vi "Perspective Calibration Example.vi"() -> ()   [LabVIEW 2011]
doc: "Description:\nThis example illustrates the use of a calibration grid to calibrate an image for perspective distortion and converts the locations of features found in the image into the locations in the real world. The example then performs accurate measurements in real world units using these locations.\n\nThis example loads a template image of a grid that is used to calibrate a system, uses the image loaded to learn the calibration from the grid, and measures distances of a distortion template with the learned calibration information."
uses:
  <vilib>/vision/Pattern Matching.llb/IMAQ Curve Parameters.ctl
  <vilib>/vision/Calibration.llb/Error Statistics.ctl
  <vilib>/vision/Calibration.llb/Distortion Model.ctl
  <vilib>/vision/Calibration.llb/Distortion Model Types.ctl
  <vilib>/vision/Clamp.llb/Edge Polarity Type.ctl
  <vilib>/vision/NI_Vision_Development_Module.lvlib
panel:
  out "Part Measurements":T1(array[cluster]) {"Distance (Pixels)" format="%#.2g"; "Distance (Real World)" format="%#.2g"; "Angle (Absolute)" format="%#.2g"; "Angle (Relative)" format="%#_2g"}
  out "Calibration Error Statistics":T2 {"% Distortion" format="%#.6g"; "Standard Deviation" format="%#.6g"; "Mean Error" format="%#.6g"; "Maximum Error" format="%#.6g"}
  in  "Curve Extraction Settings":T3={"Extraction Mode"=0, "Edge Threshold"=40, "Edge Filter Size"=1, "Min Length"=10, "Row Search Step Size"=5, "Col Search Step Size"=5, "Max Endpoint Gap"=5, "Closed"=FALSE, "Subpixel"=FALSE} {"Extraction Mode" items=["Normal", "Uniform Regions"]; "Edge Filter Size" items=["Fine", "Normal", "Contour Tracing"]; "Max Endpoint Gap" min=0; "Col Search Step Size" min=1 max=255 step=1; "Row Search Step Size" min=1 max=255 step=1; "Min Length" min=0; "Edge Threshold" min=1 max=350 step=1}
  in  "Tab Control":T4(tab)
  out "Display 4":T5(plugin-control)
  out "Display 1":T5(plugin-control)
  out "Display 2":T5(plugin-control)
  out "Display 3":T5(plugin-control)
  out "Parts Image Path":path
  out "Calibration Grid Path":path
  # "This example demonstrates how to use a calibration grid to learn the distortion model for a camera and image acquisition setup, and how to learn a perspective calibration using a polynomial model.\n\nThe calibration is used to calibrate an image acquired with the same setup, and then locate and measure parts in the image."
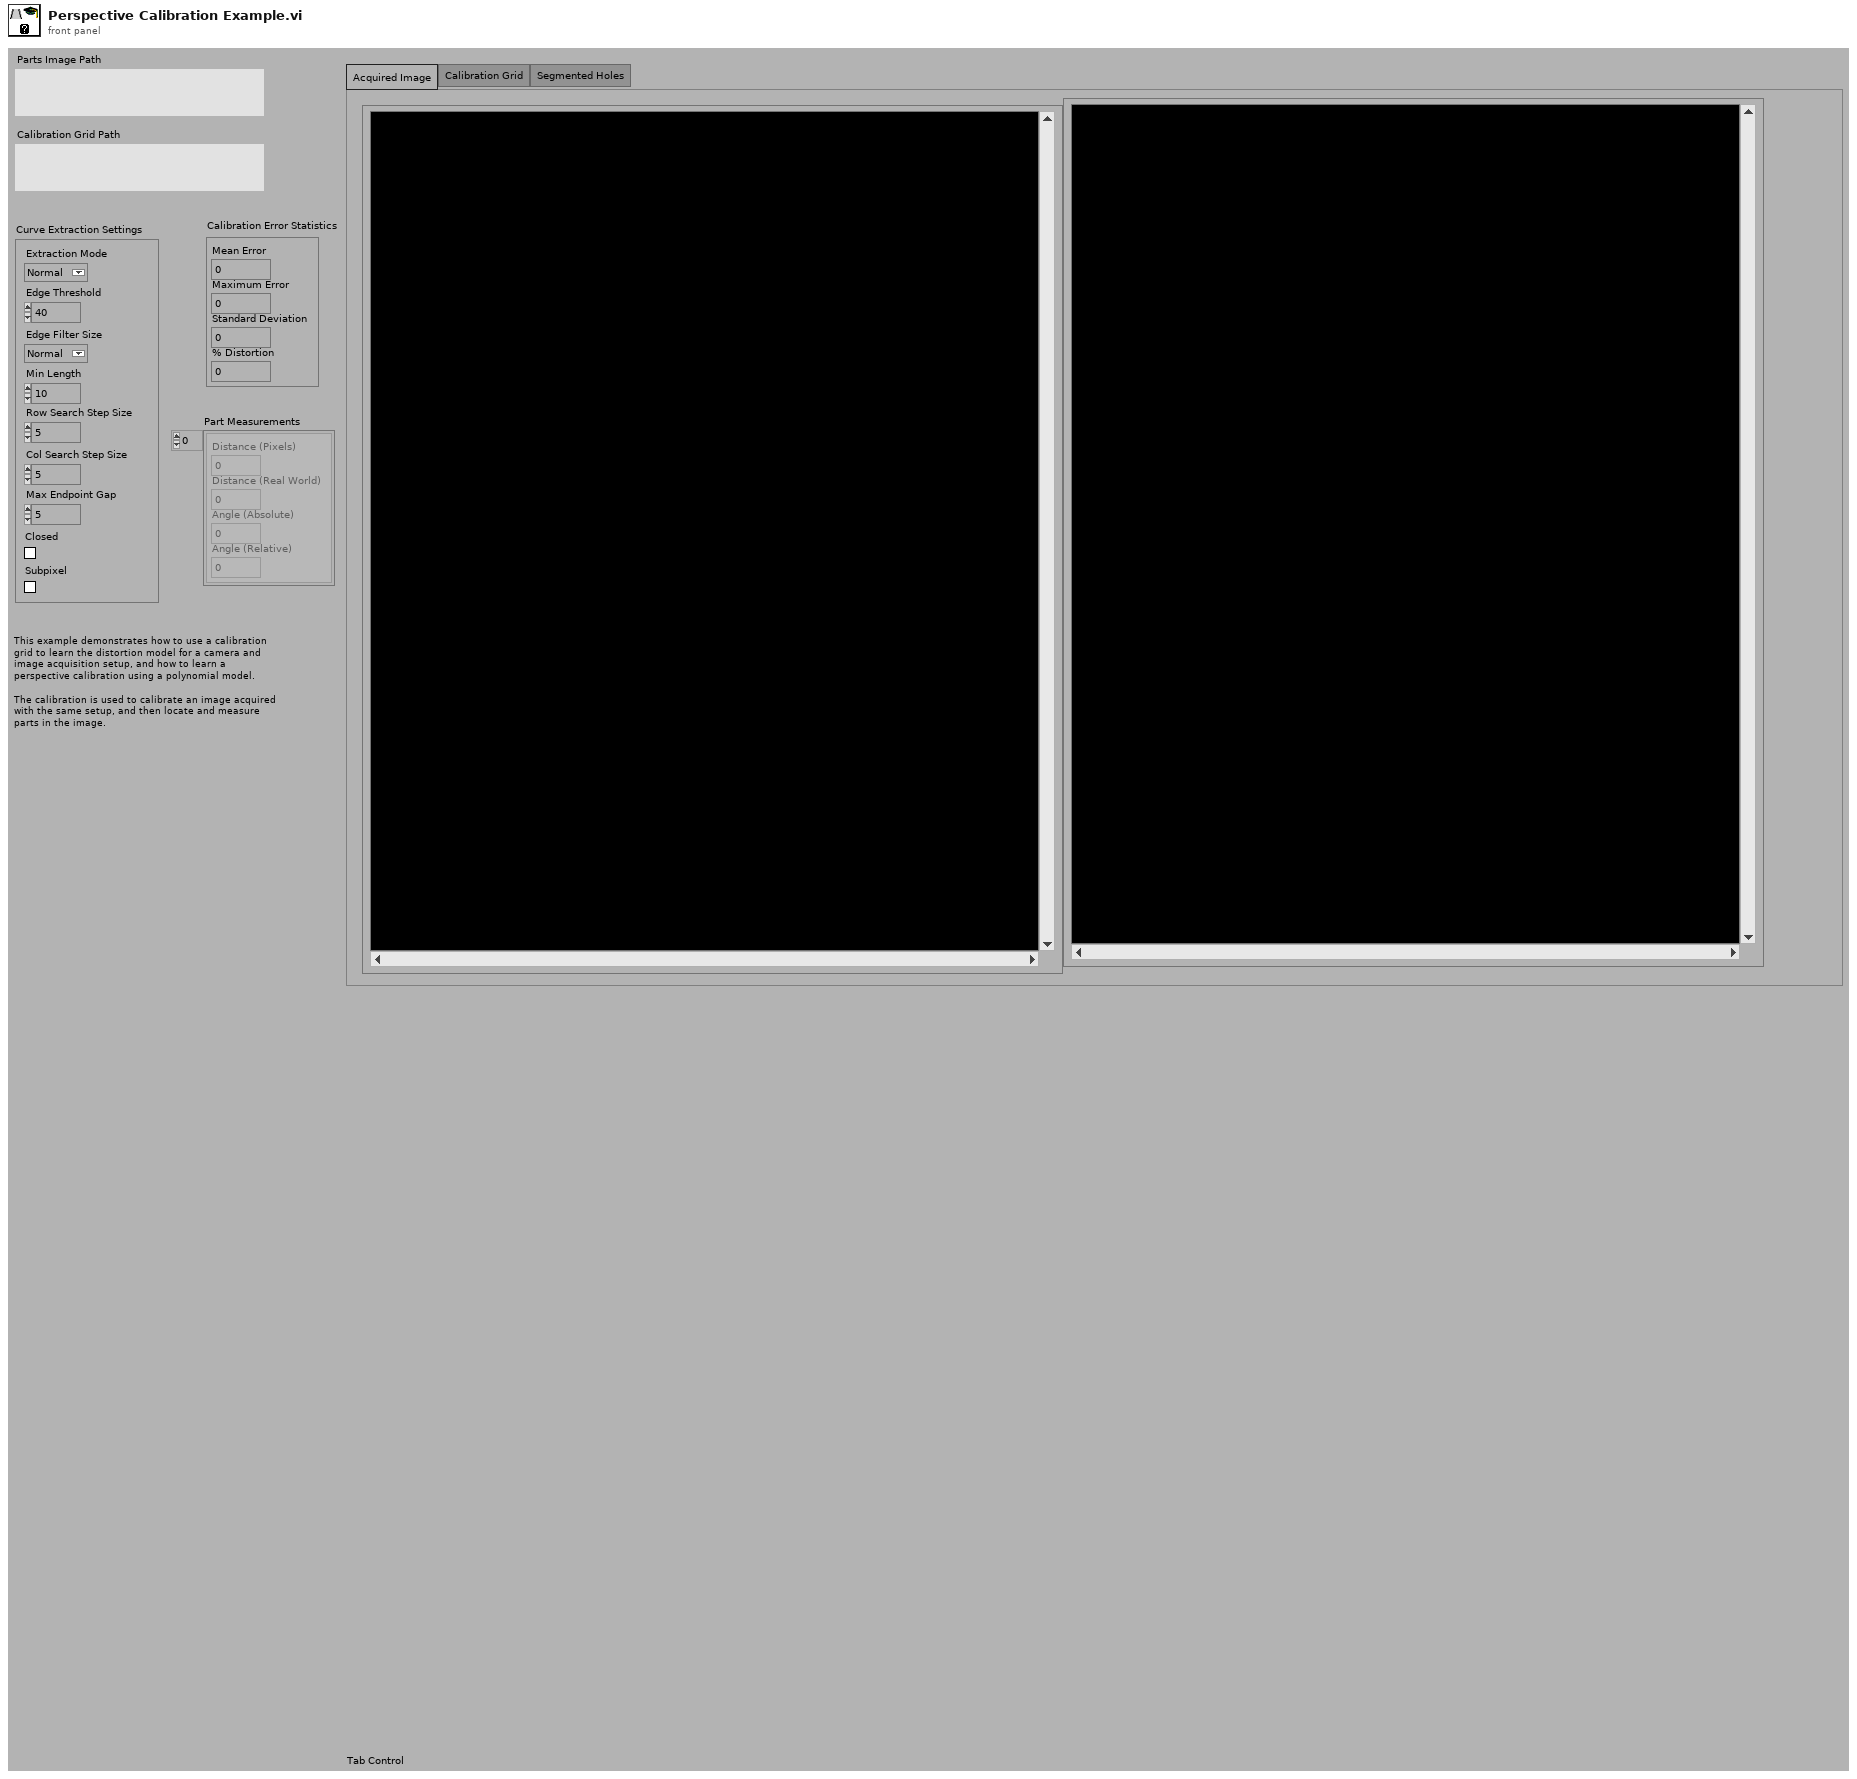
[diagram p1: front panel]
types:
  T1 = cluster{"Distance (Pixels)":dbl, "Distance (Real World)":dbl, "Angle (Absolute)":dbl, "Angle (Relative)":dbl}[]
  T2 = typedef "Error Statistics.ctl" = cluster{"Mean Error":dbl, "Maximum Error":dbl, "Standard Deviation":dbl, "% Distortion":dbl}
  T3 = typedef "IMAQ Curve Parameters.ctl" = cluster{"Extraction Mode":u32, "Edge Threshold":i32, "Edge Filter Size":u32, "Min Length":i32, "Row Search Step Size":i32, "Col Search Step Size":i32, "Max Endpoint Gap":i32, "Closed":bool, "Subpixel":bool}
  T4 = enum32{"Acquired Image", "Calibration Grid", "Segmented Holes"}
  T5 = typedef "IMAQ Image.ctl" = refnum<image>
  T6 = typedef "Distortion Model.ctl" = cluster{"Distortion Model":T7, "Polynomial Model Setup":cluster{"Radial Coefficient":u32, "Tangential Coefficients ":bool}}
  T7 = typedef "Distortion Model Types.ctl" = i32
  T8 = typedef "Particle Parameters" = i32
  T9 = cluster{"Measurement Parameter":T8, "Range Lower Value":dbl, "Range Upper Value":dbl, "Range":bool, "Measurement Type":bool}[]
  T10 = typedef "Image Unit" = enum32{"Undefined", "Angström", "Micrometer", "Millimeter", "Centimeter", "Meter", "Kilometer", "Microinch", "Inch", "Feet", "Nautical miles", "Standard miles", "Steps"}
  T11 = typedef "Calibration Reference Points.ctl" = cluster{"Pixel Coordinates":cluster{"X":dbl, "Y":dbl}[], "Real World Coordinates":cluster{"X":dbl, "Y":dbl}[], "Unit":T10, "Image Size":cluster{"X":u32, "Y":u32}}
  T12 = cluster{"Area":dbl, "Number of Holes":dbl, "Bounding Rect":cluster{"Left":dbl, "Top":dbl, "Right":dbl, "Bottom":dbl}, "Center of Mass":cluster{"X":dbl, "Y":dbl}, "Orientation":dbl, "Dimensions":cluster{"Width":dbl, "Height":dbl}}[]
  T13 = cluster{"Show Search Area":bool, "Show Curves":bool, "Show Clamp Locations":bool, "Show Result":bool, "Search Area Color":u32, "Curves Color":u32, "Clamp Locations Color":u32, "Result Color":u32, "Overlay Group Name":string}
  T14 = typedef "Edge Polarity Type.ctl" = u32
  T15 = cluster{"Angle Range (+/-)":dbl, "Edge Polarity":cluster{"Start":T14, "End":T14}}
  T16 = typedef "ROI Descriptor" = cluster{"Global Rectangle":i32[], "Contours":cluster{"ID":enum32{"External", "Internal"}, "Type":u32, "Coordinates":i32[]}[]}
  T17 = cluster{"Distance (Pixels)":dbl, "Distance (Real World)":dbl, "Angle (Absolute)":dbl, "Angle (Relative)":dbl}
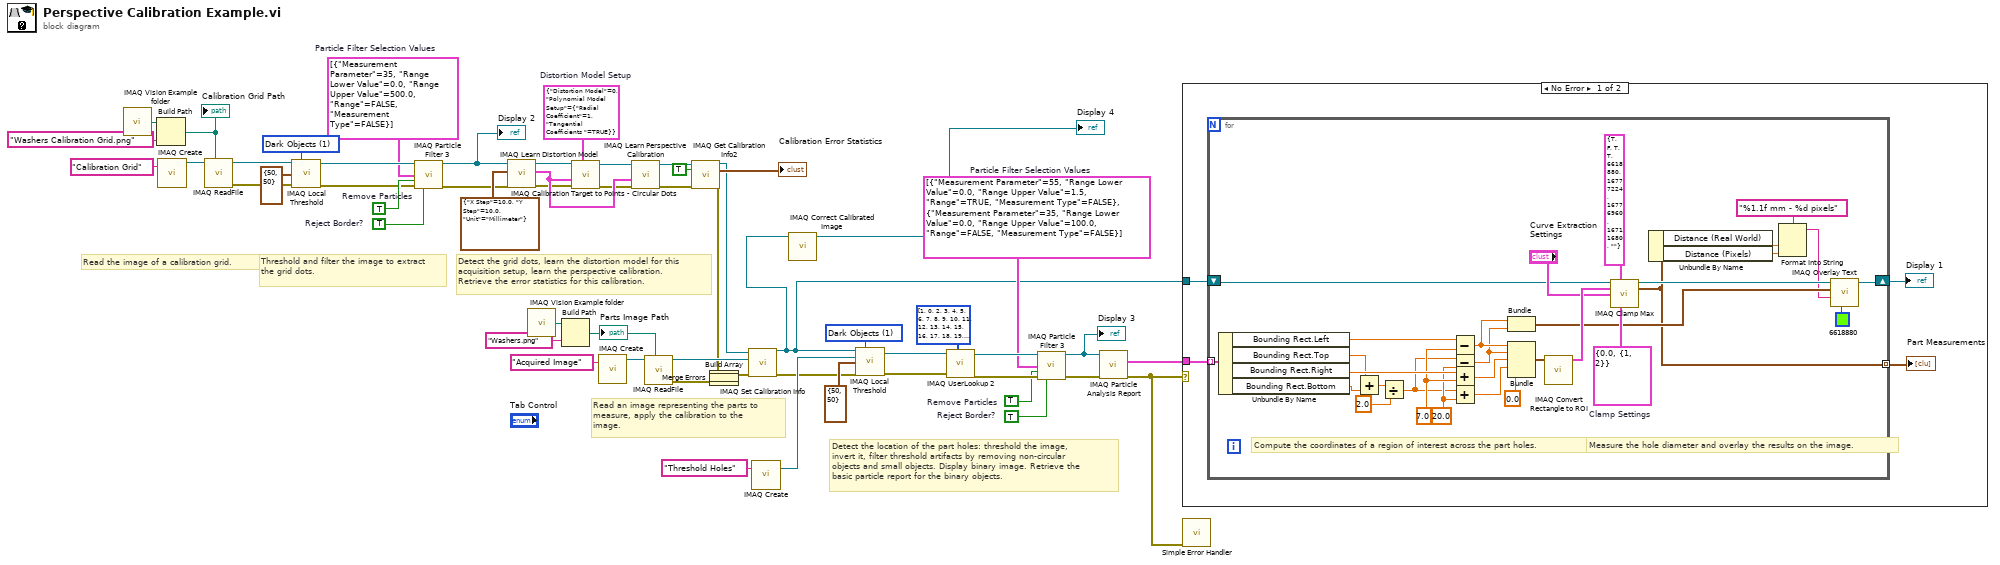
[diagram p0: block diagram]
diagram:
  w11 = TRUE  # Remove Particles
  w12 = TRUE  # Reject Border?
  w27 = T6 {"Distortion Model"=0, "Polynomial Model Setup"={"Radial Coefficient"=1, "Tangential Coefficients "=TRUE}}  # Distortion Model Setup
  w28 = T9 [{"Measurement Parameter"=35, "Range Lower Value"=0.0, "Range Upper Value"=500.0, "Range"=FALSE, "Measurement Type"=FALSE}]  # Particle Filter Selection Values
  w32 = TRUE  # Remove Particles
  w31 = TRUE  # Reject Border?
  w42 = u32 1 items=["Bright Objects", "Dark Objects"] ("Look For (Bright Objects)")
  w44 = T9 [{"Measurement Parameter"=55, "Range Lower Value"=0.0, "Range Upper Value"=1.5, "Range"=TRUE, "Measurement Type"=FALSE}, {"Measurement Parameter"=35, "Range Lower Value"=0.0, "Range Upper Value"=100.0, "Range"=FALSE, "Measurement Type"=FALSE}]  # Particle Filter Selection Values
  w51 = u32 1 items=["Bright Objects", "Dark Objects"] ("Look For (Bright Objects)")
  # "Detect the location of the part holes: threshold the image, invert it, filter threshold artifacts by removing non-circular objects and small objects. Display binary image. Retrieve the basic particle report for the binary objects."
  # "Read an image representing the parts to measure, apply the calibration to the image."
  # "Detect the grid dots, learn the distortion model for this acquisition setup, learn the perspective calibration. Retrieve the error statistics for this calibration."
  # "Threshold and filter the image to extract the grid dots."
  # "Read the image of a calibration grid."
  n1 = call "IMAQ Vision Example folder.vi"() -> ("Example Image Path"=w7:path)  [unwired: 1 out]
  n2 = Build Path(base path=w7, name or relative path="Washers Calibration Grid.png") -> (appended path=w6:path)
  "Calibration Grid Path" <- w6
  n3 = call "IMAQ Create"("Image Name"="Calibration Grid") -> ("New Image"=w55:T5)  [unwired: 3 in, 2 out]
  n4 = call "IMAQ ReadFile"("File Path"=w6, "Image"=w55) -> ("error out"=w26:errorcluster, "Image Out"=w41:T5)  [unwired: 3 in, 5 out]
  n5 = call "IMAQ Local Threshold"("Image Src"=w41, "Look For (Bright Objects)"=w42, "Window Size (32x32)"=cluster{"SizeX":i32, "SizeY":i32} {"SizeX"=50, "SizeY"=50}, "error in (no error)"=w26) -> ("Image Dst Out"=w30:T5, "error out"=w25:errorcluster)  [unwired: 4 in, 6 out]
  n6 = call "IMAQ Particle Filter 3"("Image Src"=w30, "Selection Values"=w28, "Keep/Remove Particles (F)"=w32, "error in (no error)"=w25, "Reject Border? (F)"=w31) -> ("Image Dst Out"=w29:T5, "error out"=w24:errorcluster)  [unwired: 4 in, 5 out]
  "Display 2" <- w29
  n7 = call "IMAQ Calibration Target to Points - Circular Dots"("error in (no error)"=w24, "Grid Descriptor"=cluster{"X Step":sgl, "Y Step":sgl, "Unit":T10} {"X Step"=10.0, "Y Step"=10.0, "Unit"=enum."Millimeter"}, "Target Image"=w29) -> ("error out"=w23:errorcluster, "Reference Points"=w38:T11, "Target Image (dup)"=w40:T5)  [unwired: 2 in, 4 out]
  n8 = call "IMAQ Vision Example folder.vi"() -> ("Example Image Path"=w5:path)  [unwired: 1 out]
  n9 = Build Path(base path=w5, name or relative path="Washers.png") -> (appended path=w3:path)
  "Parts Image Path" <- w3
  n10 = call "IMAQ Learn Distortion Model"("Distortion Model Setup"=w27, "error in (no error)"=w23, "Reference Points"=w38, "Calibration Template Image"=w40) -> ("error out"=w22:errorcluster, "Calibration Template Image Out"=w39:T5)  [unwired: 2 in, 4 out]
  n11 = call "IMAQ Create"("Image Name"="Acquired Image") -> ("New Image"=w54:T5)  [unwired: 3 in, 2 out]
  n12 = call "IMAQ Learn Perspective Calibration"("error in (no error)"=w22, "Reference Points"=w38, "Calibration Template Image"=w39) -> ("error out"=w21:errorcluster, "Calibration Template Image Out"=w37:T5)  [unwired: 1 in, 6 out]
  n13 = call "IMAQ ReadFile"("File Path"=w3, "Image"=w54) -> ("error out"=w20:errorcluster, "Image Out"=w47:T5)  [unwired: 3 in, 5 out]
  n14 = call "IMAQ Get Calibration Info2"("Calibration Template Image"=w37, "Return Error Information (False)"=TRUE, "error in (no error)"=w21) -> ("Calibration Template Image (duplicate)"=w33:T5, "Error Statistics"=→"Calibration Error Statistics":T2, "error out"=w19:errorcluster)  [unwired: 10 out]
  n15 = Build Array(w19, w20) -> (w9:errorcluster[])
  n16 = Merge Errors(w9) -> (w18:errorcluster)
  n17 = call "IMAQ Set Calibration Info"("error in (no error)"=w18, "Image Dst"=w47, "Image Src"=w33) -> ("error out"=w17:errorcluster, "Calibrated Image"=w2:T5)  [unwired: 1 in, 6 out]
  n18 = call "IMAQ Create"("Image Name"="Threshold Holes") -> ("New Image"=w52:T5)  [unwired: 3 in, 2 out]
  n19 = call "IMAQ Correct Calibrated Image"("Image Src"=w2) -> ("Corrected Image"=→"Display 4":T5)  [unwired: 9 in, 1 out]
  n20 = call "IMAQ Local Threshold"("Image Src"=w2, "Look For (Bright Objects)"=w51, "Image Dst"=w52, "Window Size (32x32)"=cluster{"SizeX":i32, "SizeY":i32} {"SizeX"=50, "SizeY"=50}, "error in (no error)"=w17) -> ("Image Dst Out"=w49:T5, "error out"=w16:errorcluster)  [unwired: 3 in, 6 out]
  n21 = call "IMAQ UserLookup 2"("Image Src"=w49, "Lookup Table"=i32[] [1, 0, 2, 3, 4, 5, 6, 7, 8, 9, 10, 11, 12, 13, 14, 15, 16, 17, 18, 19, 20, 21, 22, 23, 24, 25, 26, 27, 28, 29, 30, 31, 32, 33, 34, 35, 36, 37, 38, 39, 40, 41, 42, 43, 44, 45, 46, 47, 48, 49, 50, 51, 52, 53, 54, 55, 56, 57, 58, 59, 60, 61, 62, 63, 64, 65, 66, 67, 68, 69, 70, 71, 72, 73, 74, 75, 76, 77, 78, 79, 80, 81, 82, 83, 84, 85, 86, 87, 88, 89, 90, 91, 92, 93, 94, 95, 96, 97, 98, 99, 100, 101, 102, 103, 104, 105, 106, 107, 108, 109, 110, 111, 112, 113, 114, 115, 116, 117, 118, 119, 120, 121, 122, 123, 124, 125, 126, 127, 128, 129, 130, 131, 132, 133, 134, 135, 136, 137, 138, 139, 140, 141, 142, 143, 144, 145, 146, 147, 148, 149, 150, 151, 152, 153, 154, 155, 156, 157, 158, 159, 160, 161, 162, 163, 164, 165, 166, 167, 168, 169, 170, 171, 172, 173, 174, 175, 176, 177, 178, 179, 180, 181, 182, 183, 184, 185, 186, 187, 188, 189, 190, 191, 192, 193, 194, 195, 196, 197, 198, 199, 200, 201, 202, 203, 204, 205, 206, 207, 208, 209, 210, 211, 212, 213, 214, 215, 216, 217, 218, 219, 220, 221, 222, 223, 224, 225, 226, 227, 228, 229, 230, 231, 232, 233, 234, 235, 236, 237, 238, 239, 240, 241, 242, 243, 244, 245, 246, 247, 248, 249, 250, 251, 252, 253, 254, 255], "error in (no error)"=w16) -> ("Image Dst Out"=w45:T5, "error out"=w15:errorcluster)  [unwired: 2 in, 2 out]
  n22 = call "IMAQ Particle Filter 3"("Image Src"=w45, "Selection Values"=w44, "Keep/Remove Particles (F)"=w11, "error in (no error)"=w15, "Reject Border? (F)"=w12) -> ("Image Dst Out"=w10:T5, "error out"=w14:errorcluster)  [unwired: 4 in, 5 out]
  "Display 3" <- w10
  n23 = call "IMAQ Particle Analysis Report"("error in (no error)"=w14, "Image"=w10) -> ("error out"=w13:errorcluster, "Particle Reports (Pixels)"=w48:T12)  [unwired: 1 in, 7 out]
  n24 = case shown="No Error" w13 {
    tunnel: w48 -> [w61 _]
    tunnel: w2 -> [w59 _]
    frame No Error {
      n25 = for {
        tunnel: w61 -> [w91] mode=indexing
        shift-right: [w71] -> w60
        shift-left: w59 -> [w73]
        tunnel: [w62] -> w58 mode=indexing
        w79 = T15 {"Angle Range (+/-)"=0.0, "Edge Polarity"={"Start"=1, "End"=2}}  # Clamp Settings
        w83 = 20.0 ("y")
        w88 = 7.0 ("y")
        # "Measure the hole diameter and overlay the results on the image."
        # "Compute the coordinates of a region of interest across the part holes."
        n26 = Unbundle By Name(w91) -> ("Bounding Rect.Left"=w76:dbl, "Bounding Rect.Top"=w64:dbl, "Bounding Rect.Right"=w89:dbl, "Bounding Rect.Bottom"=w63:dbl)
        n27 = Add(x=w64, y=w63) -> (x+y=w85:dbl)
        n28 = Divide(x=w85, y=2.0) -> (x/y=w74:dbl)
        n29 = Subtract(x=w76, y=w88) -> (x-y=w70:dbl)
        n30 = Subtract(x=w74, y=w83) -> (x-y=w69:dbl)
        n31 = Add(x=w89, y=w88) -> (x+y=w87:dbl)
        n32 = Add(x=w74, y=w83) -> (x+y=w86:dbl)
        n33 = Bundle(w70, w69) -> (w68:cluster{dbl, dbl})  [unwired: 1 out]
        n34 = Bundle(w70, w69, w87, w86, "y"=0.0) -> (w90:cluster{dbl, dbl, dbl, dbl, "y":dbl})  [unwired: 1 out]
        n35 = call "IMAQ Convert Rectangle to ROI"("Rectangle"=w90) -> ("ROI Descriptor"=w81:T16)  [unwired: 1 in, 8 out]
        n36 = call "IMAQ Clamp Max"("Source Image"=w73, "Overlay Settings"=T13 {"Show Search Area"=TRUE, "Show Curves"=FALSE, "Show Clamp Locations"=TRUE, "Show Result"=TRUE, "Search Area Color"=6618880, "Curves Color"=16777224, "Clamp Locations Color"=16776960, "Result Color"=16711680, "Overlay Group Name"=""}, "ROI Descriptor"=w81, "Curve Extraction Settings"="Curve Extraction Settings", "Clamp Settings"=w79) -> ("Image Out"=w72:T5, "Clamp Results"=w62:T17)  [unwired: 2 in, 7 out]
        n37 = Unbundle By Name(w62) -> ("Distance (Real World)"=w67:dbl, "Distance (Pixels)"=w66:dbl)
        n38 = Format Into String(format string="%1.1f mm - %d pixels", w67, w66) -> (resulting string=w65:string)  [unwired: 2 in, 1 out]
        n39 = call "IMAQ Overlay Text"("Text Color (black)"=u32 6618880, "String"=w65, "Origin"=w68, "Image"=w72) -> ("Image Out"=w71:T5)  [unwired: 4 in, 3 out]
      }
      "Display 1" <- w60
      "Part Measurements" <- w58
    }
    frame Error {
    }
  }
  n40 = call <vilib>:"Simple Error Handler.vi"("error in (no error)"=w13) -> ()  [unwired: 1 in, 8 out]
